vi "Nest Msg Send.vi"(8 "Alias":string, 9 "Priority?":bool, 10 "Msg":refnum<class "Msg.lvclass">, 11 "Self Actor in":refnum<class "Self Actor.lvclass">) -> (0 "error out":errorcluster)   [LabVIEW 2021, in "LVCAM.lvlib" / "Self Actor.lvclass"]
uses:
  Self Actor.lvclass
  Msg/Msg.lvclass
  Self Actor.lvclass/Self Actor.ctl
  Msg Q/Msg Q.lvclass
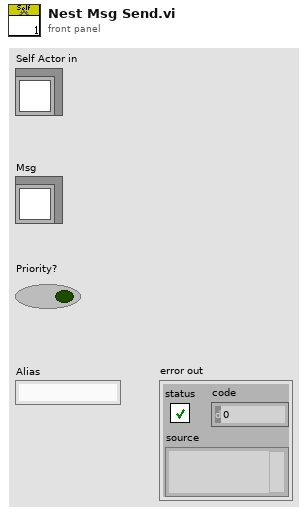
[diagram p1: front panel]
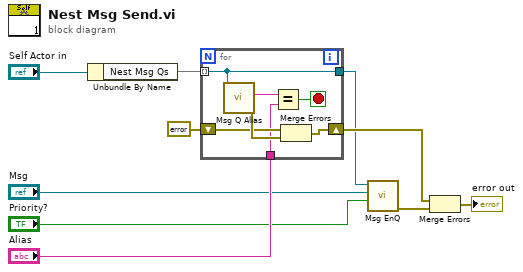
[diagram p0: block diagram]
diagram:
  n1 = Unbundle By Name("Self Actor in") -> ("Nest Msg Qs"=w9:set{refnum<class "Msg Q.lvclass">})
  n2 = for {
    tunnel: w9 -> [w16] mode=indexing
    tunnel: "Alias" -> [w11]
    tunnel: [w16] -> w4
    shift-right: [w14] -> w6
    shift-left: errorcluster {"status"=FALSE, "code"=0, "source"=""} ("error out") -> [w13]
    stop <- w17 stop-if-true
    n3 = call "Msg Q Alias.vi"("Msg Q in"=w16) -> ("error out"=w15:errorcluster, "Msg Q Alias"=w12:string)  [unwired: 9 in]
    n4 = Equal?(x=w12, y=w11) -> (x = y?=w17:bool)
    n5 = Merge Errors(w13, w15) -> (w14:errorcluster)
  }
  n6 = call "Msg EnQ.vi"("Priority?"="Priority?", "Msg"="Msg", "Msg Q in"=w4) -> ("error out"=w1:errorcluster)  [unwired: 8 in]
  n7 = Merge Errors(w6, w1) -> (→"error out":errorcluster)
